vi "Handle Command.vi"(8 "error in (no error)":errorcluster, 9 "Data":variant, 10 "Command":string, 11 "Example Instrument in":refnum<class "Example.lvclass">) -> (0 "error out":errorcluster, 1 "Processed Data":variant, 2 "Command":string, 3 "Example Instrument out":refnum<class "Example.lvclass">)   [LabVIEW 2019, in "Example.lvclass"]
uses:
  Example.lvclass
  bdcadac8-205a-486e-8dab-aa1d44b209ea.vi
  Instrument Types/VSource/Instrument.VSource.lvclass
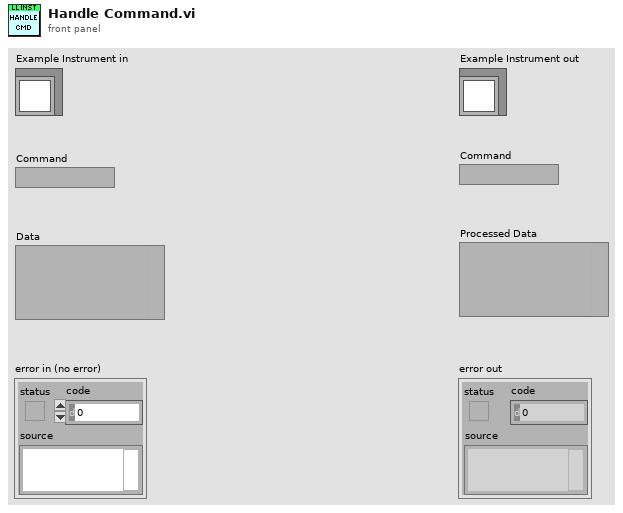
[diagram p1: front panel]
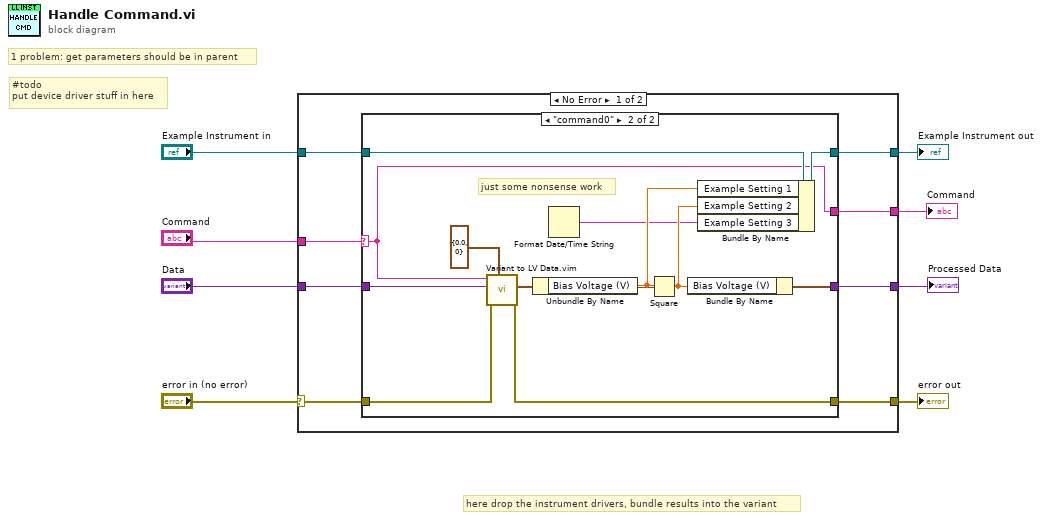
[diagram p0: block diagram]
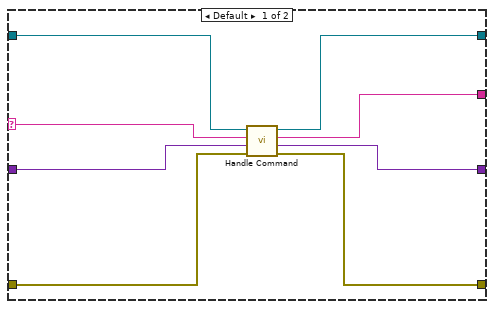
[diagram p2: hidden frame]
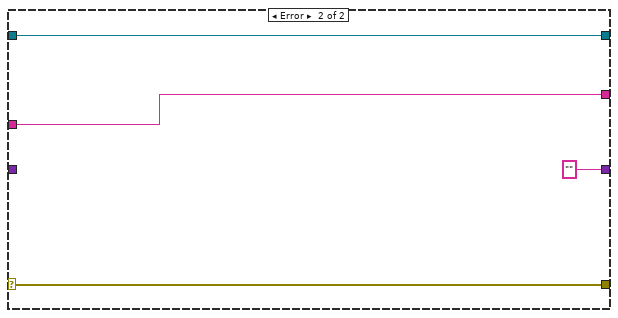
[diagram p3: hidden frame]
diagram:
  # "here drop the instrument drivers, bundle results into the variant"
  # "1 problem: get parameters should be in parent"
  # "#todo\nput device driver stuff in here"
  n1 = case shown="No Error" "error in (no error)" {
    selector: "error in (no error)" -> [w12 w40]
    tunnel: [w10 w40] -> w6
    tunnel: [w14 w39] -> w5
    tunnel: "Example Instrument in" -> [w15 w39]
    tunnel: "Command" -> [w16 w37]
    tunnel: [w13 "" ("String")] -> w3
    tunnel: "Data" -> [w11 _]
    tunnel: [w9 w37] -> w1
    frame No Error {
      n2 = case shown="\"command0\"" w16 {
        selector: w16 -> [w24 w26]
        tunnel: w15 -> [w21 w34]
        tunnel: [w18 w33] -> w14
        tunnel: [w20 w36] -> w13
        tunnel: w12 -> [w22 w29]
        tunnel: w11 -> [w23 w25]
        tunnel: [w19 w28] -> w10
        tunnel: [w17 w26] -> w9
        frame Default {
          n3 = call-parent "Handle Command.vi"("error in (no error)"=w22, "Data"=w23, "Command"=w24, "Instrument in"=w21) -> ("error out"=w19:errorcluster, "Processed Data"=w20:variant, "Command"=w17:string, "Instrument out"=w18:refnum<class "Example.lvclass">)  [unwired: 4 in]
        }
        frame "command0" {
          # "just some nonsense work"
          n4 = call "Variant to LV Data.vim"("type"=cluster{"Bias Voltage (V)":dbl, "Channel":i32} {"Bias Voltage (V)"=0.0, "Channel"=0} ("output cluster"), "error in (no error)"=w29, "Data in"=w25, "Command"=w26) -> ("error out"=w28:errorcluster, "Data out"=w27:cluster{"Bias Voltage (V)":dbl, "Channel":i32})  [unwired: 5 in, 1 out]
          n5 = Unbundle By Name(w27) -> ("Bias Voltage (V)"=w31:dbl)
          n6 = Format Date/Time String() -> (date/time string=w30:string)  [unwired: 3 in]
          n7 = Square(x=w31) -> (x^2=w32:dbl)
          n8 = Bundle By Name(cluster=w27, "Bias Voltage (V)"=w32) -> (w36:cluster{"Bias Voltage (V)":dbl, "Channel":i32})
          n9 = Bundle By Name(cluster=w34, "Example Setting 1"=w31, "Example Setting 2"=w32, "Example Setting 3"=w30) -> (w33:refnum<class "Example.lvclass">)
        }
      }
    }
    frame Error {
    }
  }
  "error out" <- w6
  "Example Instrument out" <- w5
  "Command" <- w1
  "Processed Data" <- w3
